vi "输入数据解析.vi"(0 "单个参数补充":dbl, 1 "从板号":dbl=1.0, 2 "主板二维码":string="BNET01", 3 "从板二维码":string="BNET01", 5 "主板引用":refnum<vi>, 7 "从板引用":refnum<vi>, 9 "主板选项":string="三级故障阀值", 11 "枚举":enum16{"主板", "从板"}(ring), 12 "快换":bool caption="快换写入") -> (4 "输出数组":dbl[][](array[numeric]), 6 "数组长度":dbl[](array[numeric]), 8 "循环次数":i32, 10 "命令":u32, 14 "名称":string[](array[string]), 15 "命令序号":u32[](array[numeric]))   [LabVIEW 2013] (continued)
                n6183 = property class="Tbl (严格)"(reference=w15998) -> ("Value"=w15996:string[][])  [unwired: 1 in, 2 out]
                n6184 = Multiply(x=w16001, y=2.0) -> (x*y=w15999:dbl)
                n6185 = Index Array(array=w15996, index (col)=1 ("禁用的索引 (列)")) -> (element=w16012:string[])  [unwired: 1 in]
                n6186 = Multiply(x=w16001, y=11.0) -> (x*y=w16002:dbl)
                n6187 = Divide(x=w15999, y=2.0) -> (x/y=w16004:dbl)
                n6188 = Multiply(x=w15999, y=1.5) -> (x*y=w16015:dbl)
                n6189 = Array Subset(array=w16012, index=w16002, length=w15999) -> (w16010:string[])
                n6190 = Round Toward +Infinity(x=w16004) -> (ceil(x): smallest int >= x=w16003:dbl)
                n6191 = Round Toward +Infinity(x=w16015) -> (ceil(x): smallest int >= x=w16007:dbl)
                n6192 = Fract/Exp String To Number(string=w16010) -> (number=w16013:dbl[])  [unwired: 4 out]
                n6193 = for {
                  N: w16003 -> [_]
                  tunnel: w16013 -> [w16039]
                  tunnel: [w16017] -> w16016 mode=indexing
                  i -> [w16038]
                  w16029 = 256.0 ("y")
                  n6194 = Multiply(x=w16038, y=2) -> (x*y=w16036:i32)
                  n6195 = Increment(x=w16036) -> (x+1=w16035:i32)
                  n6196 = Index Array(array=w16039, index #1=w16036, index #2=w16035) -> (element #1=w16030:dbl)  [unwired: 1 out]
                  n6197 = Quotient & Remainder(x=w16030, y=w16029) -> (x-y*floor(x/y)=w16018:dbl, floor(x/y)=w16026:dbl)
                  n6198 = Quotient & Remainder(x=w16030, y=w16029) -> (x-y*floor(x/y)=w16027:dbl, floor(x/y)=w16028:dbl)
                  n6199 = call "二进制解析-8.6.vi"("索引"=4, "数值"=w16026) -> ("低位子数组"=w16022:i32[])  [unwired: 3 out]
                  n6200 = call "二进制解析-8.6.vi"("索引"=4, "数值"=w16028) -> ("低位子数组"=w16025:i32[])  [unwired: 3 out]
                  n6201 = call "二进制解析-8.6.vi"("索引"=4, "数值"=w16027) -> ("低位子数组"=w16023:i32[], "高位子数组"=w16024:i32[])  [unwired: 2 out]
                  n6202 = Insert Into Array(array=w16025, new element=w16024) -> (w16032:i32[])  [unwired: 1 in]
                  n6203 = Insert Into Array(array=w16023, new element=w16022) -> (w16021:i32[])  [unwired: 1 in]
                  n6204 = call "数值二进制转十进制-8.6.vi"("子数组"=w16021) -> ("十进制数值"=w16019:i32)  [unwired: 4 out]
                  n6205 = call "数值二进制转十进制-8.6.vi"("子数组"=w16032) -> ("十进制数值"=w16020:i32)  [unwired: 4 out]
                  n6206 = Build Array(w16020, w16019, w16018) -> (w16017:dbl[])
                }
                n6207 = Reshape Array(w16016, w16007) -> (w16006:dbl[])
              }
              frame 4 {
                n6208 = Unbundle By Name(w16041) -> ("项目信息 2"=w16042:refnum<vi>)
                n6209 = property class="Tbl (严格)"(reference=w16042) -> ("Value"=w16040:string[][])  [unwired: 1 in, 2 out]
                n6210 = Index Array(array=w16040, index (col)=1 ("禁用的索引 (列)")) -> (element=w16047:string[])  [unwired: 1 in]
                n6211 = Multiply(x=w16046, y=6.0) -> (x*y=w16044:dbl)
                n6212 = Array Subset(array=w16047, index=0 ("索引"), length=w16044) -> (w16048:string[])
                n6213 = Fract/Exp String To Number(string=w16048) -> (number=w16045:dbl[])  [unwired: 4 out]
              }
            }
          }
        }
        frame "风机开启温差" {
          n6214 = for {
            N: 1 -> [_]
            tunnel: w16058 -> [w16062]
            tunnel: [w16065] -> w16057 mode=indexing
            tunnel: [w16064] -> w16056 mode=indexing
            tunnel: [w16063] -> w16055 mode=indexing
            tunnel: w16054 -> [w16061]
            i -> [w16066]
            n6215 = case shown="0, 默认" w16066 {
              tunnel: w16061 -> [w16081 w16087 w16128 w16172 w16216]
              tunnel: w16062 -> [_ w16091 w16132 w16176 w16221]
              tunnel: [w16069 w16092 w16137 w16181 w16220] -> w16065
              tunnel: [7.0 w16093 w16138 w16182 w16219] -> w16064
              tunnel: [u32 5 ("命令序号") u32 2 ("命令序号") u32 3 ("命令序号") u32 4 ("命令序号") u32 1 ("命令序号")] -> w16063
              frame 0, Default {
                w16067 = 255 ("高字节1")
                n6216 = Unbundle By Name(w16081) -> ("加热控制参数"=w16082:refnum<vi>)
                n6217 = property class="Clust (严格)"(reference=w16082) -> ("Value"=w16080:T5)  [unwired: 1 in, 2 out]
                n6218 = Unbundle(w16080) -> ("风机开启温度"=w16075:dbl, "风机关闭温度"=w16074:dbl, "加热开启温度"=w16071:dbl, "加热关闭温度"=w16070:dbl, "风机开启温差"=w16068:dbl)  [unwired: 2 out]
                n6219 = call "输入分辨率计算-EV05.vi"("1字节?"=TRUE, "数值 2"=w16070, "数值"=w16071, "偏移量"=-40.0, "分辨率"=1.0) -> ()  [unwired: 7 out]
                n6220 = call "输入分辨率计算-EV05.vi"("1字节?"=TRUE, "数值 2"=w16074, "数值"=w16075, "偏移量"=-40.0, "分辨率"=1.0) -> ()  [unwired: 7 out]
                n6221 = Build Array(w16067, w16067, w16068, w16067, w16067, w16067, w16067) -> (w16069:dbl[])
              }
              frame 1 {
                # "电压起始值"
                n6222 = Unbundle By Name(w16087) -> ("项目信息 2"=w16086:refnum<vi>)
                n6223 = property class="Tbl (严格)"(reference=w16086) -> ("Value"=w16085:string[][])  [unwired: 1 in, 2 out]
                n6224 = Index Array(array=w16085, index (col)=1 ("禁用的索引 (列)")) -> (element=w16099:string[])  [unwired: 1 in]
                n6225 = Multiply(x=w16091, y=6.0) -> (x*y=w16095:dbl)
                n6226 = Divide(x=w16091, y=2.0) -> (x/y=w16089:dbl)
                n6227 = Multiply(x=w16091, y=1.5) -> (x*y=w16102:dbl)
                n6228 = Array Subset(array=w16099, index=w16095, length=w16091) -> (w16097:string[])
                n6229 = Round Toward +Infinity(x=w16089) -> (ceil(x): smallest int >= x=w16088:dbl)
                n6230 = Round Toward +Infinity(x=w16102) -> (ceil(x): smallest int >= x=w16093:dbl)
                n6231 = Fract/Exp String To Number(string=w16097) -> (number=w16100:dbl[])  [unwired: 4 out]
                n6232 = for {
                  N: w16088 -> [_]
                  tunnel: w16100 -> [w16126]
                  tunnel: [w16104] -> w16103 mode=indexing
                  i -> [w16125]
                  w16116 = 256.0 ("y")
                  n6233 = Multiply(x=w16125, y=2) -> (x*y=w16123:i32)
                  n6234 = Increment(x=w16123) -> (x+1=w16122:i32)
                  n6235 = Index Array(array=w16126, index #1=w16123, index #2=w16122) -> (element #1=w16117:dbl)  [unwired: 1 out]
                  n6236 = Quotient & Remainder(x=w16117, y=w16116) -> (x-y*floor(x/y)=w16105:dbl, floor(x/y)=w16113:dbl)
                  n6237 = Quotient & Remainder(x=w16117, y=w16116) -> (x-y*floor(x/y)=w16114:dbl, floor(x/y)=w16115:dbl)
                  n6238 = call "二进制解析-8.6.vi"("索引"=4, "数值"=w16113) -> ("低位子数组"=w16109:i32[])  [unwired: 3 out]
                  n6239 = call "二进制解析-8.6.vi"("索引"=4, "数值"=w16115) -> ("低位子数组"=w16112:i32[])  [unwired: 3 out]
                  n6240 = call "二进制解析-8.6.vi"("索引"=4, "数值"=w16114) -> ("低位子数组"=w16110:i32[], "高位子数组"=w16111:i32[])  [unwired: 2 out]
                  n6241 = Insert Into Array(array=w16112, new element=w16111) -> (w16119:i32[])  [unwired: 1 in]
                  n6242 = Insert Into Array(array=w16110, new element=w16109) -> (w16108:i32[])  [unwired: 1 in]
                  n6243 = call "数值二进制转十进制-8.6.vi"("子数组"=w16108) -> ("十进制数值"=w16106:i32)  [unwired: 4 out]
                  n6244 = call "数值二进制转十进制-8.6.vi"("子数组"=w16119) -> ("十进制数值"=w16107:i32)  [unwired: 4 out]
                  n6245 = Build Array(w16107, w16106, w16105) -> (w16104:dbl[])
                }
                n6246 = Reshape Array(w16103, w16093) -> (w16092:dbl[])
              }
              frame 2 {
                # "电压起始值"
                n6247 = Unbundle By Name(w16128) -> ("项目信息 2"=w16129:refnum<vi>)
                n6248 = property class="Tbl (严格)"(reference=w16129) -> ("Value"=w16127:string[][])  [unwired: 1 in, 2 out]
                n6249 = Multiply(x=w16132, y=5.0) -> (x*y=w16130:dbl)
                n6250 = Index Array(array=w16127, index (col)=1 ("禁用的索引 (列)")) -> (element=w16143:string[])  [unwired: 1 in]
                n6251 = Multiply(x=w16132, y=7.0) -> (x*y=w16133:dbl)
                n6252 = Divide(x=w16130, y=2.0) -> (x/y=w16135:dbl)
                n6253 = Multiply(x=w16130, y=1.5) -> (x*y=w16146:dbl)
                n6254 = Array Subset(array=w16143, index=w16133, length=w16130) -> (w16141:string[])
                n6255 = Round Toward +Infinity(x=w16135) -> (ceil(x): smallest int >= x=w16134:dbl)
                n6256 = Round Toward +Infinity(x=w16146) -> (ceil(x): smallest int >= x=w16138:dbl)
                n6257 = Fract/Exp String To Number(string=w16141) -> (number=w16144:dbl[])  [unwired: 4 out]
                n6258 = for {
                  N: w16134 -> [_]
                  tunnel: w16144 -> [w16170]
                  tunnel: [w16148] -> w16147 mode=indexing
                  i -> [w16169]
                  w16160 = 256.0 ("y")
                  n6259 = Multiply(x=w16169, y=2) -> (x*y=w16167:i32)
                  n6260 = Increment(x=w16167) -> (x+1=w16166:i32)
                  n6261 = Index Array(array=w16170, index #1=w16167, index #2=w16166) -> (element #1=w16161:dbl)  [unwired: 1 out]
                  n6262 = Quotient & Remainder(x=w16161, y=w16160) -> (x-y*floor(x/y)=w16149:dbl, floor(x/y)=w16157:dbl)
                  n6263 = Quotient & Remainder(x=w16161, y=w16160) -> (x-y*floor(x/y)=w16158:dbl, floor(x/y)=w16159:dbl)
                  n6264 = call "二进制解析-8.6.vi"("索引"=4, "数值"=w16157) -> ("低位子数组"=w16153:i32[])  [unwired: 3 out]
                  n6265 = call "二进制解析-8.6.vi"("索引"=4, "数值"=w16159) -> ("低位子数组"=w16156:i32[])  [unwired: 3 out]
                  n6266 = call "二进制解析-8.6.vi"("索引"=4, "数值"=w16158) -> ("低位子数组"=w16154:i32[], "高位子数组"=w16155:i32[])  [unwired: 2 out]
                  n6267 = Insert Into Array(array=w16156, new element=w16155) -> (w16163:i32[])  [unwired: 1 in]
                  n6268 = Insert Into Array(array=w16154, new element=w16153) -> (w16152:i32[])  [unwired: 1 in]
                  n6269 = call "数值二进制转十进制-8.6.vi"("子数组"=w16152) -> ("十进制数值"=w16150:i32)  [unwired: 4 out]
                  n6270 = call "数值二进制转十进制-8.6.vi"("子数组"=w16163) -> ("十进制数值"=w16151:i32)  [unwired: 4 out]
                  n6271 = Build Array(w16151, w16150, w16149) -> (w16148:dbl[])
                }
                n6272 = Reshape Array(w16147, w16138) -> (w16137:dbl[])
              }
              frame 3 {
                # "电压起始值"
                n6273 = Unbundle By Name(w16172) -> ("项目信息 2"=w16173:refnum<vi>)
                n6274 = property class="Tbl (严格)"(reference=w16173) -> ("Value"=w16171:string[][])  [unwired: 1 in, 2 out]
                n6275 = Multiply(x=w16176, y=2.0) -> (x*y=w16174:dbl)
                n6276 = Index Array(array=w16171, index (col)=1 ("禁用的索引 (列)")) -> (element=w16187:string[])  [unwired: 1 in]
                n6277 = Multiply(x=w16176, y=11.0) -> (x*y=w16177:dbl)
                n6278 = Divide(x=w16174, y=2.0) -> (x/y=w16179:dbl)
                n6279 = Multiply(x=w16174, y=1.5) -> (x*y=w16190:dbl)
                n6280 = Array Subset(array=w16187, index=w16177, length=w16174) -> (w16185:string[])
                n6281 = Round Toward +Infinity(x=w16179) -> (ceil(x): smallest int >= x=w16178:dbl)
                n6282 = Round Toward +Infinity(x=w16190) -> (ceil(x): smallest int >= x=w16182:dbl)
                n6283 = Fract/Exp String To Number(string=w16185) -> (number=w16188:dbl[])  [unwired: 4 out]
                n6284 = for {
                  N: w16178 -> [_]
                  tunnel: w16188 -> [w16214]
                  tunnel: [w16192] -> w16191 mode=indexing
                  i -> [w16213]
                  w16204 = 256.0 ("y")
                  n6285 = Multiply(x=w16213, y=2) -> (x*y=w16211:i32)
                  n6286 = Increment(x=w16211) -> (x+1=w16210:i32)
                  n6287 = Index Array(array=w16214, index #1=w16211, index #2=w16210) -> (element #1=w16205:dbl)  [unwired: 1 out]
                  n6288 = Quotient & Remainder(x=w16205, y=w16204) -> (x-y*floor(x/y)=w16193:dbl, floor(x/y)=w16201:dbl)
                  n6289 = Quotient & Remainder(x=w16205, y=w16204) -> (x-y*floor(x/y)=w16202:dbl, floor(x/y)=w16203:dbl)
                  n6290 = call "二进制解析-8.6.vi"("索引"=4, "数值"=w16201) -> ("低位子数组"=w16197:i32[])  [unwired: 3 out]
                  n6291 = call "二进制解析-8.6.vi"("索引"=4, "数值"=w16203) -> ("低位子数组"=w16200:i32[])  [unwired: 3 out]
                  n6292 = call "二进制解析-8.6.vi"("索引"=4, "数值"=w16202) -> ("低位子数组"=w16198:i32[], "高位子数组"=w16199:i32[])  [unwired: 2 out]
                  n6293 = Insert Into Array(array=w16200, new element=w16199) -> (w16207:i32[])  [unwired: 1 in]
                  n6294 = Insert Into Array(array=w16198, new element=w16197) -> (w16196:i32[])  [unwired: 1 in]
                  n6295 = call "数值二进制转十进制-8.6.vi"("子数组"=w16196) -> ("十进制数值"=w16194:i32)  [unwired: 4 out]
                  n6296 = call "数值二进制转十进制-8.6.vi"("子数组"=w16207) -> ("十进制数值"=w16195:i32)  [unwired: 4 out]
                  n6297 = Build Array(w16195, w16194, w16193) -> (w16192:dbl[])
                }
                n6298 = Reshape Array(w16191, w16182) -> (w16181:dbl[])
              }
              frame 4 {
                n6299 = Unbundle By Name(w16216) -> ("项目信息 2"=w16217:refnum<vi>)
                n6300 = property class="Tbl (严格)"(reference=w16217) -> ("Value"=w16215:string[][])  [unwired: 1 in, 2 out]
                n6301 = Index Array(array=w16215, index (col)=1 ("禁用的索引 (列)")) -> (element=w16222:string[])  [unwired: 1 in]
                n6302 = Multiply(x=w16221, y=6.0) -> (x*y=w16219:dbl)
                n6303 = Array Subset(array=w16222, index=0 ("索引"), length=w16219) -> (w16223:string[])
                n6304 = Fract/Exp String To Number(string=w16223) -> (number=w16220:dbl[])  [unwired: 4 out]
              }
            }
          }
        }
        frame "风机关闭温差" {
          n6305 = for {
            N: 1 -> [_]
            tunnel: w16233 -> [w16237]
            tunnel: [w16240] -> w16232 mode=indexing
            tunnel: [w16239] -> w16231 mode=indexing
            tunnel: [w16238] -> w16230 mode=indexing
            tunnel: w16229 -> [w16236]
            i -> [w16241]
            n6306 = case shown="0, 默认" w16241 {
              tunnel: w16236 -> [w16256 w16262 w16303 w16347 w16391]
              tunnel: w16237 -> [_ w16266 w16307 w16351 w16396]
              tunnel: [w16244 w16267 w16312 w16356 w16395] -> w16240
              tunnel: [7.0 w16268 w16313 w16357 w16394] -> w16239
              tunnel: [u32 5 ("命令序号") u32 2 ("命令序号") u32 3 ("命令序号") u32 4 ("命令序号") u32 1 ("命令序号")] -> w16238
              frame 0, Default {
                w16242 = 255 ("高字节1")
                n6307 = Unbundle By Name(w16256) -> ("加热控制参数"=w16257:refnum<vi>)
                n6308 = property class="Clust (严格)"(reference=w16257) -> ("Value"=w16255:T5)  [unwired: 1 in, 2 out]
                n6309 = Unbundle(w16255) -> ("风机开启温度"=w16250:dbl, "风机关闭温度"=w16249:dbl, "加热开启温度"=w16246:dbl, "加热关闭温度"=w16245:dbl, "风机关闭温差"=w16243:dbl)  [unwired: 2 out]
                n6310 = call "输入分辨率计算-EV05.vi"("1字节?"=TRUE, "数值 2"=w16245, "数值"=w16246, "偏移量"=-40.0, "分辨率"=1.0) -> ()  [unwired: 7 out]
                n6311 = call "输入分辨率计算-EV05.vi"("1字节?"=TRUE, "数值 2"=w16249, "数值"=w16250, "偏移量"=-40.0, "分辨率"=1.0) -> ()  [unwired: 7 out]
                n6312 = Build Array(w16242, w16242, w16242, w16243, w16242, w16242, w16242) -> (w16244:dbl[])
              }
              frame 1 {
                # "电压起始值"
                n6313 = Unbundle By Name(w16262) -> ("项目信息 2"=w16261:refnum<vi>)
                n6314 = property class="Tbl (严格)"(reference=w16261) -> ("Value"=w16260:string[][])  [unwired: 1 in, 2 out]
                n6315 = Index Array(array=w16260, index (col)=1 ("禁用的索引 (列)")) -> (element=w16274:string[])  [unwired: 1 in]
                n6316 = Multiply(x=w16266, y=6.0) -> (x*y=w16270:dbl)
                n6317 = Divide(x=w16266, y=2.0) -> (x/y=w16264:dbl)
                n6318 = Multiply(x=w16266, y=1.5) -> (x*y=w16277:dbl)
                n6319 = Array Subset(array=w16274, index=w16270, length=w16266) -> (w16272:string[])
                n6320 = Round Toward +Infinity(x=w16264) -> (ceil(x): smallest int >= x=w16263:dbl)
                n6321 = Round Toward +Infinity(x=w16277) -> (ceil(x): smallest int >= x=w16268:dbl)
                n6322 = Fract/Exp String To Number(string=w16272) -> (number=w16275:dbl[])  [unwired: 4 out]
                n6323 = for {
                  N: w16263 -> [_]
                  tunnel: w16275 -> [w16301]
                  tunnel: [w16279] -> w16278 mode=indexing
                  i -> [w16300]
                  w16291 = 256.0 ("y")
                  n6324 = Multiply(x=w16300, y=2) -> (x*y=w16298:i32)
                  n6325 = Increment(x=w16298) -> (x+1=w16297:i32)
                  n6326 = Index Array(array=w16301, index #1=w16298, index #2=w16297) -> (element #1=w16292:dbl)  [unwired: 1 out]
                  n6327 = Quotient & Remainder(x=w16292, y=w16291) -> (x-y*floor(x/y)=w16280:dbl, floor(x/y)=w16288:dbl)
                  n6328 = Quotient & Remainder(x=w16292, y=w16291) -> (x-y*floor(x/y)=w16289:dbl, floor(x/y)=w16290:dbl)
                  n6329 = call "二进制解析-8.6.vi"("索引"=4, "数值"=w16288) -> ("低位子数组"=w16284:i32[])  [unwired: 3 out]
                  n6330 = call "二进制解析-8.6.vi"("索引"=4, "数值"=w16290) -> ("低位子数组"=w16287:i32[])  [unwired: 3 out]
                  n6331 = call "二进制解析-8.6.vi"("索引"=4, "数值"=w16289) -> ("低位子数组"=w16285:i32[], "高位子数组"=w16286:i32[])  [unwired: 2 out]
                  n6332 = Insert Into Array(array=w16287, new element=w16286) -> (w16294:i32[])  [unwired: 1 in]
                  n6333 = Insert Into Array(array=w16285, new element=w16284) -> (w16283:i32[])  [unwired: 1 in]
                  n6334 = call "数值二进制转十进制-8.6.vi"("子数组"=w16283) -> ("十进制数值"=w16281:i32)  [unwired: 4 out]
                  n6335 = call "数值二进制转十进制-8.6.vi"("子数组"=w16294) -> ("十进制数值"=w16282:i32)  [unwired: 4 out]
                  n6336 = Build Array(w16282, w16281, w16280) -> (w16279:dbl[])
                }
                n6337 = Reshape Array(w16278, w16268) -> (w16267:dbl[])
              }
              frame 2 {
                # "电压起始值"
                n6338 = Unbundle By Name(w16303) -> ("项目信息 2"=w16304:refnum<vi>)
                n6339 = property class="Tbl (严格)"(reference=w16304) -> ("Value"=w16302:string[][])  [unwired: 1 in, 2 out]
                n6340 = Multiply(x=w16307, y=5.0) -> (x*y=w16305:dbl)
                n6341 = Index Array(array=w16302, index (col)=1 ("禁用的索引 (列)")) -> (element=w16318:string[])  [unwired: 1 in]
                n6342 = Multiply(x=w16307, y=7.0) -> (x*y=w16308:dbl)
                n6343 = Divide(x=w16305, y=2.0) -> (x/y=w16310:dbl)
                n6344 = Multiply(x=w16305, y=1.5) -> (x*y=w16321:dbl)
                n6345 = Array Subset(array=w16318, index=w16308, length=w16305) -> (w16316:string[])
                n6346 = Round Toward +Infinity(x=w16310) -> (ceil(x): smallest int >= x=w16309:dbl)
                n6347 = Round Toward +Infinity(x=w16321) -> (ceil(x): smallest int >= x=w16313:dbl)
                n6348 = Fract/Exp String To Number(string=w16316) -> (number=w16319:dbl[])  [unwired: 4 out]
                n6349 = for {
                  N: w16309 -> [_]
                  tunnel: w16319 -> [w16345]
                  tunnel: [w16323] -> w16322 mode=indexing
                  i -> [w16344]
                  w16335 = 256.0 ("y")
                  n6350 = Multiply(x=w16344, y=2) -> (x*y=w16342:i32)
                  n6351 = Increment(x=w16342) -> (x+1=w16341:i32)
                  n6352 = Index Array(array=w16345, index #1=w16342, index #2=w16341) -> (element #1=w16336:dbl)  [unwired: 1 out]
                  n6353 = Quotient & Remainder(x=w16336, y=w16335) -> (x-y*floor(x/y)=w16324:dbl, floor(x/y)=w16332:dbl)
                  n6354 = Quotient & Remainder(x=w16336, y=w16335) -> (x-y*floor(x/y)=w16333:dbl, floor(x/y)=w16334:dbl)
                  n6355 = call "二进制解析-8.6.vi"("索引"=4, "数值"=w16332) -> ("低位子数组"=w16328:i32[])  [unwired: 3 out]
                  n6356 = call "二进制解析-8.6.vi"("索引"=4, "数值"=w16334) -> ("低位子数组"=w16331:i32[])  [unwired: 3 out]
                  n6357 = call "二进制解析-8.6.vi"("索引"=4, "数值"=w16333) -> ("低位子数组"=w16329:i32[], "高位子数组"=w16330:i32[])  [unwired: 2 out]
                  n6358 = Insert Into Array(array=w16331, new element=w16330) -> (w16338:i32[])  [unwired: 1 in]
                  n6359 = Insert Into Array(array=w16329, new element=w16328) -> (w16327:i32[])  [unwired: 1 in]
                  n6360 = call "数值二进制转十进制-8.6.vi"("子数组"=w16327) -> ("十进制数值"=w16325:i32)  [unwired: 4 out]
                  n6361 = call "数值二进制转十进制-8.6.vi"("子数组"=w16338) -> ("十进制数值"=w16326:i32)  [unwired: 4 out]
                  n6362 = Build Array(w16326, w16325, w16324) -> (w16323:dbl[])
                }
                n6363 = Reshape Array(w16322, w16313) -> (w16312:dbl[])
              }
              frame 3 {
                # "电压起始值"
                n6364 = Unbundle By Name(w16347) -> ("项目信息 2"=w16348:refnum<vi>)
                n6365 = property class="Tbl (严格)"(reference=w16348) -> ("Value"=w16346:string[][])  [unwired: 1 in, 2 out]
                n6366 = Multiply(x=w16351, y=2.0) -> (x*y=w16349:dbl)
                n6367 = Index Array(array=w16346, index (col)=1 ("禁用的索引 (列)")) -> (element=w16362:string[])  [unwired: 1 in]
                n6368 = Multiply(x=w16351, y=11.0) -> (x*y=w16352:dbl)
                n6369 = Divide(x=w16349, y=2.0) -> (x/y=w16354:dbl)
                n6370 = Multiply(x=w16349, y=1.5) -> (x*y=w16365:dbl)
                n6371 = Array Subset(array=w16362, index=w16352, length=w16349) -> (w16360:string[])
                n6372 = Round Toward +Infinity(x=w16354) -> (ceil(x): smallest int >= x=w16353:dbl)
                n6373 = Round Toward +Infinity(x=w16365) -> (ceil(x): smallest int >= x=w16357:dbl)
                n6374 = Fract/Exp String To Number(string=w16360) -> (number=w16363:dbl[])  [unwired: 4 out]
                n6375 = for {
                  N: w16353 -> [_]
                  tunnel: w16363 -> [w16389]
                  tunnel: [w16367] -> w16366 mode=indexing
                  i -> [w16388]
                  w16379 = 256.0 ("y")
                  n6376 = Multiply(x=w16388, y=2) -> (x*y=w16386:i32)
                  n6377 = Increment(x=w16386) -> (x+1=w16385:i32)
                  n6378 = Index Array(array=w16389, index #1=w16386, index #2=w16385) -> (element #1=w16380:dbl)  [unwired: 1 out]
                  n6379 = Quotient & Remainder(x=w16380, y=w16379) -> (x-y*floor(x/y)=w16368:dbl, floor(x/y)=w16376:dbl)
                  n6380 = Quotient & Remainder(x=w16380, y=w16379) -> (x-y*floor(x/y)=w16377:dbl, floor(x/y)=w16378:dbl)
                  n6381 = call "二进制解析-8.6.vi"("索引"=4, "数值"=w16376) -> ("低位子数组"=w16372:i32[])  [unwired: 3 out]
                  n6382 = call "二进制解析-8.6.vi"("索引"=4, "数值"=w16378) -> ("低位子数组"=w16375:i32[])  [unwired: 3 out]
                  n6383 = call "二进制解析-8.6.vi"("索引"=4, "数值"=w16377) -> ("低位子数组"=w16373:i32[], "高位子数组"=w16374:i32[])  [unwired: 2 out]
                  n6384 = Insert Into Array(array=w16375, new element=w16374) -> (w16382:i32[])  [unwired: 1 in]
                  n6385 = Insert Into Array(array=w16373, new element=w16372) -> (w16371:i32[])  [unwired: 1 in]
                  n6386 = call "数值二进制转十进制-8.6.vi"("子数组"=w16371) -> ("十进制数值"=w16369:i32)  [unwired: 4 out]
                  n6387 = call "数值二进制转十进制-8.6.vi"("子数组"=w16382) -> ("十进制数值"=w16370:i32)  [unwired: 4 out]
                  n6388 = Build Array(w16370, w16369, w16368) -> (w16367:dbl[])
                }
                n6389 = Reshape Array(w16366, w16357) -> (w16356:dbl[])
              }
              frame 4 {
                n6390 = Unbundle By Name(w16391) -> ("项目信息 2"=w16392:refnum<vi>)
                n6391 = property class="Tbl (严格)"(reference=w16392) -> ("Value"=w16390:string[][])  [unwired: 1 in, 2 out]
                n6392 = Index Array(array=w16390, index (col)=1 ("禁用的索引 (列)")) -> (element=w16397:string[])  [unwired: 1 in]
                n6393 = Multiply(x=w16396, y=6.0) -> (x*y=w16394:dbl)
                n6394 = Array Subset(array=w16397, index=0 ("索引"), length=w16394) -> (w16398:string[])
                n6395 = Fract/Exp String To Number(string=w16398) -> (number=w16395:dbl[])  [unwired: 4 out]
              }
            }
          }
        }
        frame "加热关闭温差" {
          n6396 = for {
            N: 1 -> [_]
            tunnel: w16408 -> [w16412]
            tunnel: [w16415] -> w16407 mode=indexing
            tunnel: [w16414] -> w16406 mode=indexing
            tunnel: [w16413] -> w16405 mode=indexing
            tunnel: w16404 -> [w16411]
            i -> [w16416]
            n6397 = case shown="0, 默认" w16416 {
              tunnel: w16411 -> [w16431 w16437 w16478 w16522 w16566]
              tunnel: w16412 -> [_ w16441 w16482 w16526 w16571]
              tunnel: [w16419 w16442 w16487 w16531 w16570] -> w16415
              tunnel: [7.0 w16443 w16488 w16532 w16569] -> w16414
              tunnel: [u32 5 ("命令序号") u32 2 ("命令序号") u32 3 ("命令序号") u32 4 ("命令序号") u32 1 ("命令序号")] -> w16413
              frame 0, Default {
                w16418 = 255 ("高字节1")
                n6398 = Unbundle By Name(w16431) -> ("加热控制参数"=w16432:refnum<vi>)
                n6399 = property class="Clust (严格)"(reference=w16432) -> ("Value"=w16430:T5)  [unwired: 1 in, 2 out]
                n6400 = Unbundle(w16430) -> ("风机开启温度"=w16425:dbl, "风机关闭温度"=w16424:dbl, "加热开启温度"=w16421:dbl, "加热关闭温度"=w16420:dbl, "加热关闭温差"=w16417:dbl)  [unwired: 2 out]
                n6401 = call "输入分辨率计算-EV05.vi"("1字节?"=TRUE, "数值 2"=w16420, "数值"=w16421, "偏移量"=-40.0, "分辨率"=1.0) -> ()  [unwired: 7 out]
                n6402 = call "输入分辨率计算-EV05.vi"("1字节?"=TRUE, "数值 2"=w16424, "数值"=w16425, "偏移量"=-40.0, "分辨率"=1.0) -> ()  [unwired: 7 out]
                n6403 = Build Array(w16418, w16418, w16418, w16418, w16418, w16418, w16417) -> (w16419:dbl[])
              }
              frame 1 {
                # "电压起始值"
                n6404 = Unbundle By Name(w16437) -> ("项目信息 2"=w16436:refnum<vi>)
                n6405 = property class="Tbl (严格)"(reference=w16436) -> ("Value"=w16435:string[][])  [unwired: 1 in, 2 out]
                n6406 = Index Array(array=w16435, index (col)=1 ("禁用的索引 (列)")) -> (element=w16449:string[])  [unwired: 1 in]
                n6407 = Multiply(x=w16441, y=6.0) -> (x*y=w16445:dbl)
                n6408 = Divide(x=w16441, y=2.0) -> (x/y=w16439:dbl)
                n6409 = Multiply(x=w16441, y=1.5) -> (x*y=w16452:dbl)
                n6410 = Array Subset(array=w16449, index=w16445, length=w16441) -> (w16447:string[])
                n6411 = Round Toward +Infinity(x=w16439) -> (ceil(x): smallest int >= x=w16438:dbl)
                n6412 = Round Toward +Infinity(x=w16452) -> (ceil(x): smallest int >= x=w16443:dbl)
                n6413 = Fract/Exp String To Number(string=w16447) -> (number=w16450:dbl[])  [unwired: 4 out]
                n6414 = for {
                  N: w16438 -> [_]
                  tunnel: w16450 -> [w16476]
                  tunnel: [w16454] -> w16453 mode=indexing
                  i -> [w16475]
                  w16466 = 256.0 ("y")
                  n6415 = Multiply(x=w16475, y=2) -> (x*y=w16473:i32)
                  n6416 = Increment(x=w16473) -> (x+1=w16472:i32)
                  n6417 = Index Array(array=w16476, index #1=w16473, index #2=w16472) -> (element #1=w16467:dbl)  [unwired: 1 out]
                  n6418 = Quotient & Remainder(x=w16467, y=w16466) -> (x-y*floor(x/y)=w16455:dbl, floor(x/y)=w16463:dbl)
                  n6419 = Quotient & Remainder(x=w16467, y=w16466) -> (x-y*floor(x/y)=w16464:dbl, floor(x/y)=w16465:dbl)
                  n6420 = call "二进制解析-8.6.vi"("索引"=4, "数值"=w16463) -> ("低位子数组"=w16459:i32[])  [unwired: 3 out]
                  n6421 = call "二进制解析-8.6.vi"("索引"=4, "数值"=w16465) -> ("低位子数组"=w16462:i32[])  [unwired: 3 out]
                  n6422 = call "二进制解析-8.6.vi"("索引"=4, "数值"=w16464) -> ("低位子数组"=w16460:i32[], "高位子数组"=w16461:i32[])  [unwired: 2 out]
                  n6423 = Insert Into Array(array=w16462, new element=w16461) -> (w16469:i32[])  [unwired: 1 in]
                  n6424 = Insert Into Array(array=w16460, new element=w16459) -> (w16458:i32[])  [unwired: 1 in]
                  n6425 = call "数值二进制转十进制-8.6.vi"("子数组"=w16458) -> ("十进制数值"=w16456:i32)  [unwired: 4 out]
                  n6426 = call "数值二进制转十进制-8.6.vi"("子数组"=w16469) -> ("十进制数值"=w16457:i32)  [unwired: 4 out]
                  n6427 = Build Array(w16457, w16456, w16455) -> (w16454:dbl[])
                }
                n6428 = Reshape Array(w16453, w16443) -> (w16442:dbl[])
              }
              frame 2 {
                # "电压起始值"
                n6429 = Unbundle By Name(w16478) -> ("项目信息 2"=w16479:refnum<vi>)
                n6430 = property class="Tbl (严格)"(reference=w16479) -> ("Value"=w16477:string[][])  [unwired: 1 in, 2 out]
                n6431 = Multiply(x=w16482, y=5.0) -> (x*y=w16480:dbl)
                n6432 = Index Array(array=w16477, index (col)=1 ("禁用的索引 (列)")) -> (element=w16493:string[])  [unwired: 1 in]
                n6433 = Multiply(x=w16482, y=7.0) -> (x*y=w16483:dbl)
                n6434 = Divide(x=w16480, y=2.0) -> (x/y=w16485:dbl)
                n6435 = Multiply(x=w16480, y=1.5) -> (x*y=w16496:dbl)
                n6436 = Array Subset(array=w16493, index=w16483, length=w16480) -> (w16491:string[])
                n6437 = Round Toward +Infinity(x=w16485) -> (ceil(x): smallest int >= x=w16484:dbl)
                n6438 = Round Toward +Infinity(x=w16496) -> (ceil(x): smallest int >= x=w16488:dbl)
                n6439 = Fract/Exp String To Number(string=w16491) -> (number=w16494:dbl[])  [unwired: 4 out]
                n6440 = for {
                  N: w16484 -> [_]
                  tunnel: w16494 -> [w16520]
                  tunnel: [w16498] -> w16497 mode=indexing
                  i -> [w16519]
                  w16510 = 256.0 ("y")
                  n6441 = Multiply(x=w16519, y=2) -> (x*y=w16517:i32)
                  n6442 = Increment(x=w16517) -> (x+1=w16516:i32)
                  n6443 = Index Array(array=w16520, index #1=w16517, index #2=w16516) -> (element #1=w16511:dbl)  [unwired: 1 out]
                  n6444 = Quotient & Remainder(x=w16511, y=w16510) -> (x-y*floor(x/y)=w16499:dbl, floor(x/y)=w16507:dbl)
                  n6445 = Quotient & Remainder(x=w16511, y=w16510) -> (x-y*floor(x/y)=w16508:dbl, floor(x/y)=w16509:dbl)
                  n6446 = call "二进制解析-8.6.vi"("索引"=4, "数值"=w16507) -> ("低位子数组"=w16503:i32[])  [unwired: 3 out]
                  n6447 = call "二进制解析-8.6.vi"("索引"=4, "数值"=w16509) -> ("低位子数组"=w16506:i32[])  [unwired: 3 out]
                  n6448 = call "二进制解析-8.6.vi"("索引"=4, "数值"=w16508) -> ("低位子数组"=w16504:i32[], "高位子数组"=w16505:i32[])  [unwired: 2 out]
                  n6449 = Insert Into Array(array=w16506, new element=w16505) -> (w16513:i32[])  [unwired: 1 in]
                  n6450 = Insert Into Array(array=w16504, new element=w16503) -> (w16502:i32[])  [unwired: 1 in]
                  n6451 = call "数值二进制转十进制-8.6.vi"("子数组"=w16502) -> ("十进制数值"=w16500:i32)  [unwired: 4 out]
                  n6452 = call "数值二进制转十进制-8.6.vi"("子数组"=w16513) -> ("十进制数值"=w16501:i32)  [unwired: 4 out]
                  n6453 = Build Array(w16501, w16500, w16499) -> (w16498:dbl[])
                }
                n6454 = Reshape Array(w16497, w16488) -> (w16487:dbl[])
              }
              frame 3 {
                # "电压起始值"
                n6455 = Unbundle By Name(w16522) -> ("项目信息 2"=w16523:refnum<vi>)
                n6456 = property class="Tbl (严格)"(reference=w16523) -> ("Value"=w16521:string[][])  [unwired: 1 in, 2 out]
                n6457 = Multiply(x=w16526, y=2.0) -> (x*y=w16524:dbl)
                n6458 = Index Array(array=w16521, index (col)=1 ("禁用的索引 (列)")) -> (element=w16537:string[])  [unwired: 1 in]
                n6459 = Multiply(x=w16526, y=11.0) -> (x*y=w16527:dbl)
                n6460 = Divide(x=w16524, y=2.0) -> (x/y=w16529:dbl)
                n6461 = Multiply(x=w16524, y=1.5) -> (x*y=w16540:dbl)
                n6462 = Array Subset(array=w16537, index=w16527, length=w16524) -> (w16535:string[])
                n6463 = Round Toward +Infinity(x=w16529) -> (ceil(x): smallest int >= x=w16528:dbl)
                n6464 = Round Toward +Infinity(x=w16540) -> (ceil(x): smallest int >= x=w16532:dbl)
                n6465 = Fract/Exp String To Number(string=w16535) -> (number=w16538:dbl[])  [unwired: 4 out]
                n6466 = for {
                  N: w16528 -> [_]
                  tunnel: w16538 -> [w16564]
                  tunnel: [w16542] -> w16541 mode=indexing
                  i -> [w16563]
                  w16554 = 256.0 ("y")
                  n6467 = Multiply(x=w16563, y=2) -> (x*y=w16561:i32)
                  n6468 = Increment(x=w16561) -> (x+1=w16560:i32)
                  n6469 = Index Array(array=w16564, index #1=w16561, index #2=w16560) -> (element #1=w16555:dbl)  [unwired: 1 out]
                  n6470 = Quotient & Remainder(x=w16555, y=w16554) -> (x-y*floor(x/y)=w16543:dbl, floor(x/y)=w16551:dbl)
                  n6471 = Quotient & Remainder(x=w16555, y=w16554) -> (x-y*floor(x/y)=w16552:dbl, floor(x/y)=w16553:dbl)
                  n6472 = call "二进制解析-8.6.vi"("索引"=4, "数值"=w16551) -> ("低位子数组"=w16547:i32[])  [unwired: 3 out]
                  n6473 = call "二进制解析-8.6.vi"("索引"=4, "数值"=w16553) -> ("低位子数组"=w16550:i32[])  [unwired: 3 out]
                  n6474 = call "二进制解析-8.6.vi"("索引"=4, "数值"=w16552) -> ("低位子数组"=w16548:i32[], "高位子数组"=w16549:i32[])  [unwired: 2 out]
                  n6475 = Insert Into Array(array=w16550, new element=w16549) -> (w16557:i32[])  [unwired: 1 in]
                  n6476 = Insert Into Array(array=w16548, new element=w16547) -> (w16546:i32[])  [unwired: 1 in]
                  n6477 = call "数值二进制转十进制-8.6.vi"("子数组"=w16546) -> ("十进制数值"=w16544:i32)  [unwired: 4 out]
                  n6478 = call "数值二进制转十进制-8.6.vi"("子数组"=w16557) -> ("十进制数值"=w16545:i32)  [unwired: 4 out]
                  n6479 = Build Array(w16545, w16544, w16543) -> (w16542:dbl[])
                }
                n6480 = Reshape Array(w16541, w16532) -> (w16531:dbl[])
              }
              frame 4 {
                n6481 = Unbundle By Name(w16566) -> ("项目信息 2"=w16567:refnum<vi>)
                n6482 = property class="Tbl (严格)"(reference=w16567) -> ("Value"=w16565:string[][])  [unwired: 1 in, 2 out]
                n6483 = Index Array(array=w16565, index (col)=1 ("禁用的索引 (列)")) -> (element=w16572:string[])  [unwired: 1 in]
                n6484 = Multiply(x=w16571, y=6.0) -> (x*y=w16569:dbl)
                n6485 = Array Subset(array=w16572, index=0 ("索引"), length=w16569) -> (w16573:string[])
                n6486 = Fract/Exp String To Number(string=w16573) -> (number=w16570:dbl[])  [unwired: 4 out]
              }
            }
          }
        }
        frame "一级故障阀值" {
          n6487 = Unbundle By Name(w16582) -> ("一级故障(从板)"=w16583:refnum<vi>)
          n6488 = property class="Clust (严格)"(reference=w16583) -> ("Value"=w16581:T8)  [unwired: 1 in, 2 out]
          n6489 = for {
            N: 7 -> [_]
            tunnel: w16581 -> [w16594]
            shift-right: [w16593] -> w16585
            shift-left: dbl[] [] -> [w16592]
            tunnel: 0.001 ("分辨率") -> [w16590]
            i -> [w16595]
            n6490 = case shown="0, 默认" w16595 {
              tunnel: w16594 -> [w16598 w16605 w16611 w16618 w16625 w16632 w16640]
              tunnel: [w16599 w16606 w16612 w16620 w16627 w16633 w16641] -> w16591
              tunnel: w16590 -> [w16596 w16603 _ _ _ _ _]
              frame 0, Default {
                # "电压过高"
                n6491 = Unbundle By Name(w16598) -> ("电压过高"=w16597:dbl)
                n6492 = call "输入分辨率计算-EV05.vi"("1字节?"=FALSE, "数值"=w16597, "分辨率"=w16596) -> ("低字节"=w16600:dbl, "高字节1"=w16601:dbl)  [unwired: 2 in, 5 out]
                n6493 = Build Array(w16601, w16600) -> (w16599:dbl[])
              }
              frame 1 {
                # "电压过低"
                n6494 = Unbundle By Name(w16605) -> ("电压过低"=w16604:dbl)
                n6495 = call "输入分辨率计算-EV05.vi"("1字节?"=FALSE, "数值"=w16604, "分辨率"=w16603) -> ("低字节"=w16607:dbl, "高字节1"=w16608:dbl)  [unwired: 2 in, 5 out]
                n6496 = Build Array(w16608, w16607) -> (w16606:dbl[])
              }
              frame 2 {
                # "电压不均衡"
                n6497 = Unbundle By Name(w16611) -> ("电压不均衡(V)"=w16610:dbl)
                n6498 = call "输入分辨率计算-EV05.vi"("1字节?"=FALSE, "数值"=w16610, "分辨率"=0.001) -> ("低字节"=w16613:dbl, "高字节1"=w16614:dbl)  [unwired: 2 in, 5 out]
                n6499 = Build Array(w16614, w16613) -> (w16612:dbl[])
              }
              frame 3 {
                # "温度过高"
                n6500 = Unbundle By Name(w16618) -> ("温度过高"=w16617:dbl)
                n6501 = call "输入分辨率计算-EV05.vi"("1字节?"=TRUE, "数值"=w16617, "偏移量"=-40.0, "分辨率"=1.0) -> ("高字节1"=w16621:dbl)  [unwired: 1 in, 6 out]
                n6502 = Build Array(w16621) -> (w16620:dbl[])
              }
              frame 4 {
                # "温度过低"
                n6503 = Unbundle By Name(w16625) -> ("温度过低"=w16624:dbl)
                n6504 = call "输入分辨率计算-EV05.vi"("1字节?"=TRUE, "数值"=w16624, "偏移量"=-40.0, "分辨率"=1.0) -> ("高字节1"=w16628:dbl)  [unwired: 1 in, 6 out]
                n6505 = Build Array(w16628) -> (w16627:dbl[])
              }
              frame 5 {
                # "温度不均衡"
                n6506 = Unbundle By Name(w16632) -> ("温度不均衡"=w16631:dbl)
                n6507 = call "输入分辨率计算-EV05.vi"("1字节?"=TRUE, "数值"=w16631, "分辨率"=1.0) -> ("高字节1"=w16634:dbl)  [unwired: 2 in, 6 out]
                n6508 = Build Array(w16634) -> (w16633:dbl[])
              }
              frame 6 {
                # "SOC过低"
                n6509 = Unbundle By Name(w16640) -> ("SOC过低"=w16639:dbl)
                n6510 = call "输入分辨率计算-EV05.vi"("1字节?"=FALSE, "数值"=w16639, "分辨率"=0.1) -> ("低字节"=w16637:dbl, "高字节1"=w16638:dbl)  [unwired: 2 in, 5 out]
                n6511 = Build Array(w16638, w16637) -> (w16641:dbl[])
              }
            }
            n6512 = Insert Into Array(array=w16592, new element=w16591) -> (w16593:dbl[])  [unwired: 1 in]
          }
          n6513 = Build Array(w16585) -> (w16584:dbl[][])
        }
        frame "电压过高" {
          n6514 = Unbundle By Name(w16648) -> ("一级故障(从板)"=w16649:refnum<vi>)
          n6515 = property class="Clust (严格)"(reference=w16649) -> ("Value"=w16647:T8)  [unwired: 1 in, 2 out]
          n6516 = for {
            N: 7 -> [_]
            tunnel: w16647 -> [w16659]
            shift-right: [w16658] -> w16651
            shift-left: dbl[] [] -> [w16657]
            i -> [w16660]
            n6517 = case shown="0, 默认" w16660 {
              tunnel: w16659 -> [w16661 w16672 w16683 w16694 w16704 w16714 w16725]
              tunnel: [w16662 w16673 w16684 w16695 w16705 w16715 w16726] -> w16656
              frame 0, Default {
                # "电压过高"
                n6518 = disable-structure shown="启用" {
                  disable-tunnel: [w16668 w16671] -> w16664
                  disable-tunnel: [w16667 w16671] -> w16663
                  disable-tunnel: w16661 -> [w16666 _]
                  frame Enabled {
                    n6519 = Unbundle By Name(w16666) -> ("电压过高"=w16665:dbl)
                    n6520 = call "输入分辨率计算-EV05.vi"("1字节?"=FALSE, "数值"=w16665, "分辨率"=0.001) -> ("低字节"=w16667:dbl, "高字节1"=w16668:dbl)  [unwired: 2 in, 5 out]
                  }
                  frame Disabled {
                    w16671 = 255 ("高字节1")
                  }
                }
                n6521 = Build Array(w16664, w16663) -> (w16662:dbl[])
              }
              frame 1 {
                # "电压过低"
                n6522 = disable-structure shown="启用" {
                  disable-tunnel: [w16679 w16682] -> w16675
                  disable-tunnel: [w16678 w16682] -> w16674
                  disable-tunnel: w16672 -> [w16677 _]
                  frame Disabled {
                    n6523 = Unbundle By Name(w16677) -> ("电压过低"=w16676:dbl)
                    n6524 = call "输入分辨率计算-EV05.vi"("1字节?"=FALSE, "数值"=w16676, "分辨率"=0.1) -> ("低字节"=w16678:dbl, "高字节1"=w16679:dbl)  [unwired: 2 in, 5 out]
                  }
                  frame Enabled {
                    w16682 = 255 ("高字节1")
                  }
                }
                n6525 = Build Array(w16675, w16674) -> (w16673:i32[])
              }
              frame 2 {
                # "电压不均衡"
                n6526 = disable-structure shown="启用" {
                  disable-tunnel: [w16690 w16693] -> w16686
                  disable-tunnel: [w16689 w16693] -> w16685
                  disable-tunnel: w16683 -> [w16688 _]
                  frame Disabled {
                    n6527 = Unbundle By Name(w16688) -> ("电压不均衡(V)"=w16687:dbl)
                    n6528 = call "输入分辨率计算-EV05.vi"("1字节?"=FALSE, "数值"=w16687, "分辨率"=0.1) -> ("低字节"=w16689:dbl, "高字节1"=w16690:dbl)  [unwired: 2 in, 5 out]
                  }
                  frame Enabled {
                    w16693 = 255 ("高字节1")
                  }
                }
                n6529 = Build Array(w16686, w16685) -> (w16684:i32[])
              }
              frame 3 {
                # "温度过高"
                n6530 = disable-structure shown="启用" {
                  disable-tunnel: [w16700 255 ("高字节1")] -> w16696
                  disable-tunnel: w16694 -> [w16698 _]
                  frame Disabled {
                    n6531 = Unbundle By Name(w16698) -> ("温度过高"=w16697:dbl)
                    n6532 = call "输入分辨率计算-EV05.vi"("1字节?"=TRUE, "数值"=w16697, "偏移量"=-40.0, "分辨率"=1.0) -> ("高字节1"=w16700:dbl)  [unwired: 1 in, 6 out]
                  }
                  frame Enabled {
                  }
                }
                n6533 = Build Array(w16696) -> (w16695:i32[])
              }
              frame 4 {
                # "温度过低"
                n6534 = disable-structure shown="启用" {
                  disable-tunnel: [w16710 255 ("高字节1")] -> w16706
                  disable-tunnel: w16704 -> [w16708 _]
                  frame Disabled {
                    n6535 = Unbundle By Name(w16708) -> ("温度过低"=w16707:dbl)
                    n6536 = call "输入分辨率计算-EV05.vi"("1字节?"=TRUE, "数值"=w16707, "偏移量"=-40.0, "分辨率"=1.0) -> ("高字节1"=w16710:dbl)  [unwired: 1 in, 6 out]
                  }
                  frame Enabled {
                  }
                }
                n6537 = Build Array(w16706) -> (w16705:i32[])
              }
              frame 5 {
                # "温度不均衡"
                n6538 = disable-structure shown="启用" {
                  disable-tunnel: [w16719 255 ("高字节1")] -> w16716
                  disable-tunnel: w16714 -> [w16718 _]
                  frame Disabled {
                    n6539 = Unbundle By Name(w16718) -> ("温度不均衡"=w16717:dbl)
                    n6540 = call "输入分辨率计算-EV05.vi"("1字节?"=TRUE, "数值"=w16717, "分辨率"=1.0) -> ("高字节1"=w16719:dbl)  [unwired: 2 in, 6 out]
                  }
                  frame Enabled {
                  }
                }
                n6541 = Build Array(w16716) -> (w16715:i32[])
              }
              frame 6 {
                # "SOC过低"
                n6542 = disable-structure shown="启用" {
                  disable-tunnel: w16725 -> [w16742 _]
                  disable-tunnel: [w16728 w16745] -> w16724
                  disable-tunnel: [w16727 w16745] -> w16723
                  frame Disabled {
                    n6543 = Unbundle By Name(w16742) -> ("SOC过低"=w16741:dbl)
                    n6544 = call "输入分辨率计算-EV05.vi"("1字节?"=FALSE, "数值"=w16741, "分辨率"=0.1) -> ("低字节"=w16730:dbl, "高字节1"=w16731:dbl)  [unwired: 2 in, 5 out]
                    n6545 = call "二进制解析-8.6.vi"("索引"=4, "数值"=0) -> ("低位子数组"=w16734:i32[])  [unwired: 3 out]
                    n6546 = call "二进制解析-8.6.vi"("索引"=4, "数值"=w16731) -> ("低位子数组"=w16737:i32[])  [unwired: 3 out]
                    n6547 = call "二进制解析-8.6.vi"("索引"=4, "数值"=w16730) -> ("低位子数组"=w16735:i32[], "高位子数组"=w16736:i32[])  [unwired: 2 out]
                    n6548 = Insert Into Array(array=w16737, new element=w16736) -> (w16739:i32[])  [unwired: 1 in]
                    n6549 = Insert Into Array(array=w16735, new element=w16734) -> (w16733:i32[])  [unwired: 1 in]
                    n6550 = call "数值二进制转十进制-8.6.vi"("子数组"=w16733) -> ("十进制数值"=w16728:i32)  [unwired: 4 out]
                    n6551 = call "数值二进制转十进制-8.6.vi"("子数组"=w16739) -> ("十进制数值"=w16727:i32)  [unwired: 4 out]
                  }
                  frame Enabled {
                    w16745 = 255 ("高字节1")
                  }
                }
                n6552 = Build Array(w16723, w16724) -> (w16726:i32[])
              }
            }
            n6553 = Insert Into Array(array=w16657, new element=w16656) -> (w16658:dbl[])  [unwired: 1 in]
          }
          n6554 = Build Array(w16651) -> (w16650:dbl[][])
        }
        frame "电压过高(2)" {
          n6555 = Unbundle By Name(w16750) -> ("二级故障(从板)"=w16751:refnum<vi>)
          n6556 = property class="Clust (严格)"(reference=w16751) -> ("Value"=w16749:T8)  [unwired: 1 in, 2 out]
          n6557 = for {
            N: 7 -> [_]
            tunnel: w16749 -> [w16761]
            shift-right: [w16760] -> w16753
            shift-left: dbl[] [] -> [w16759]
            i -> [w16762]
            n6558 = case shown="0, 默认" w16762 {
              tunnel: w16761 -> [w16763 w16774 w16785 w16796 w16806 w16816 w16827]
              tunnel: [w16764 w16775 w16786 w16797 w16807 w16817 w16828] -> w16758
              frame 0, Default {
                # "电压过高"
                n6559 = disable-structure shown="启用" {
                  disable-tunnel: [w16770 w16773] -> w16766
                  disable-tunnel: [w16769 w16773] -> w16765
                  disable-tunnel: w16763 -> [w16768 _]
                  frame Enabled {
                    n6560 = Unbundle By Name(w16768) -> ("电压过高"=w16767:dbl)
                    n6561 = call "输入分辨率计算-EV05.vi"("1字节?"=FALSE, "数值"=w16767, "分辨率"=0.001) -> ("低字节"=w16769:dbl, "高字节1"=w16770:dbl)  [unwired: 2 in, 5 out]
                  }
                  frame Disabled {
                    w16773 = 255 ("高字节1")
                  }
                }
                n6562 = Build Array(w16766, w16765) -> (w16764:dbl[])
              }
              frame 1 {
                # "电压过低"
                n6563 = disable-structure shown="启用" {
                  disable-tunnel: [w16781 w16784] -> w16777
                  disable-tunnel: [w16780 w16784] -> w16776
                  disable-tunnel: w16774 -> [w16779 _]
                  frame Disabled {
                    n6564 = Unbundle By Name(w16779) -> ("电压过低"=w16778:dbl)
                    n6565 = call "输入分辨率计算-EV05.vi"("1字节?"=FALSE, "数值"=w16778, "分辨率"=0.1) -> ("低字节"=w16780:dbl, "高字节1"=w16781:dbl)  [unwired: 2 in, 5 out]
                  }
                  frame Enabled {
                    w16784 = 255 ("高字节1")
                  }
                }
                n6566 = Build Array(w16777, w16776) -> (w16775:i32[])
              }
              frame 2 {
                # "电压不均衡"
                n6567 = disable-structure shown="启用" {
                  disable-tunnel: [w16792 w16795] -> w16788
                  disable-tunnel: [w16791 w16795] -> w16787
                  disable-tunnel: w16785 -> [w16790 _]
                  frame Disabled {
                    n6568 = Unbundle By Name(w16790) -> ("电压不均衡(V)"=w16789:dbl)
                    n6569 = call "输入分辨率计算-EV05.vi"("1字节?"=FALSE, "数值"=w16789, "分辨率"=0.1) -> ("低字节"=w16791:dbl, "高字节1"=w16792:dbl)  [unwired: 2 in, 5 out]
                  }
                  frame Enabled {
                    w16795 = 255 ("高字节1")
                  }
                }
                n6570 = Build Array(w16788, w16787) -> (w16786:i32[])
              }
              frame 3 {
                # "温度过高"
                n6571 = disable-structure shown="启用" {
                  disable-tunnel: [w16802 255 ("高字节1")] -> w16798
                  disable-tunnel: w16796 -> [w16800 _]
                  frame Disabled {
                    n6572 = Unbundle By Name(w16800) -> ("温度过高"=w16799:dbl)
                    n6573 = call "输入分辨率计算-EV05.vi"("1字节?"=TRUE, "数值"=w16799, "偏移量"=-40.0, "分辨率"=1.0) -> ("高字节1"=w16802:dbl)  [unwired: 1 in, 6 out]
                  }
                  frame Enabled {
                  }
                }
                n6574 = Build Array(w16798) -> (w16797:i32[])
              }
              frame 4 {
                # "温度过低"
                n6575 = disable-structure shown="启用" {
                  disable-tunnel: [w16812 255 ("高字节1")] -> w16808
                  disable-tunnel: w16806 -> [w16810 _]
                  frame Disabled {
                    n6576 = Unbundle By Name(w16810) -> ("温度过低"=w16809:dbl)
                    n6577 = call "输入分辨率计算-EV05.vi"("1字节?"=TRUE, "数值"=w16809, "偏移量"=-40.0, "分辨率"=1.0) -> ("高字节1"=w16812:dbl)  [unwired: 1 in, 6 out]
                  }
                  frame Enabled {
                  }
                }
                n6578 = Build Array(w16808) -> (w16807:i32[])
              }
              frame 5 {
                # "温度不均衡"
                n6579 = disable-structure shown="启用" {
                  disable-tunnel: [w16821 255 ("高字节1")] -> w16818
                  disable-tunnel: w16816 -> [w16820 _]
                  frame Disabled {
                    n6580 = Unbundle By Name(w16820) -> ("温度不均衡"=w16819:dbl)
                    n6581 = call "输入分辨率计算-EV05.vi"("1字节?"=TRUE, "数值"=w16819, "分辨率"=1.0) -> ("高字节1"=w16821:dbl)  [unwired: 2 in, 6 out]
                  }
                  frame Enabled {
                  }
                }
                n6582 = Build Array(w16818) -> (w16817:i32[])
              }
              frame 6 {
                # "SOC过低"
                n6583 = disable-structure shown="启用" {
                  disable-tunnel: w16827 -> [w16844 _]
                  disable-tunnel: [w16830 w16847] -> w16826
                  disable-tunnel: [w16829 w16847] -> w16825
                  frame Disabled {
                    n6584 = Unbundle By Name(w16844) -> ("SOC过低"=w16843:dbl)
                    n6585 = call "输入分辨率计算-EV05.vi"("1字节?"=FALSE, "数值"=w16843, "分辨率"=0.1) -> ("低字节"=w16832:dbl, "高字节1"=w16833:dbl)  [unwired: 2 in, 5 out]
                    n6586 = call "二进制解析-8.6.vi"("索引"=4, "数值"=0) -> ("低位子数组"=w16836:i32[])  [unwired: 3 out]
                    n6587 = call "二进制解析-8.6.vi"("索引"=4, "数值"=w16833) -> ("低位子数组"=w16839:i32[])  [unwired: 3 out]
                    n6588 = call "二进制解析-8.6.vi"("索引"=4, "数值"=w16832) -> ("低位子数组"=w16837:i32[], "高位子数组"=w16838:i32[])  [unwired: 2 out]
                    n6589 = Insert Into Array(array=w16839, new element=w16838) -> (w16841:i32[])  [unwired: 1 in]
                    n6590 = Insert Into Array(array=w16837, new element=w16836) -> (w16835:i32[])  [unwired: 1 in]
                    n6591 = call "数值二进制转十进制-8.6.vi"("子数组"=w16835) -> ("十进制数值"=w16830:i32)  [unwired: 4 out]
                    n6592 = call "数值二进制转十进制-8.6.vi"("子数组"=w16841) -> ("十进制数值"=w16829:i32)  [unwired: 4 out]
                  }
                  frame Enabled {
                    w16847 = 255 ("高字节1")
                  }
                }
                n6593 = Build Array(w16825, w16826) -> (w16828:i32[])
              }
            }
            n6594 = Insert Into Array(array=w16759, new element=w16758) -> (w16760:dbl[])  [unwired: 1 in]
          }
          n6595 = Build Array(w16753) -> (w16752:dbl[][])
        }
        frame "电压过高(3)" {
          n6596 = Unbundle By Name(w16852) -> ("三级故障(从板)"=w16853:refnum<vi>)
          n6597 = property class="Clust (严格)"(reference=w16853) -> ("Value"=w16851:T8)  [unwired: 1 in, 2 out]
          n6598 = for {
            N: 7 -> [_]
            tunnel: w16851 -> [w16863]
            shift-right: [w16862] -> w16855
            shift-left: dbl[] [] -> [w16861]
            i -> [w16864]
            n6599 = case shown="0, 默认" w16864 {
              tunnel: w16863 -> [w16865 w16876 w16887 w16898 w16908 w16918 w16929]
              tunnel: [w16866 w16877 w16888 w16899 w16909 w16919 w16930] -> w16860
              frame 0, Default {
                # "电压过高"
                n6600 = disable-structure shown="启用" {
                  disable-tunnel: [w16872 w16875] -> w16868
                  disable-tunnel: [w16871 w16875] -> w16867
                  disable-tunnel: w16865 -> [w16870 _]
                  frame Enabled {
                    n6601 = Unbundle By Name(w16870) -> ("电压过高"=w16869:dbl)
